vi "test - submodule case.vi"(8 "error in (no error)":errorcluster, 11 "TestCase in":refnum<class "csm-ini-variable-addon.lvclass">) -> (0 "error out":errorcluster, 3 "TestCase out":refnum<class "csm-ini-variable-addon.lvclass">)   [LabVIEW 2017, in "csm-ini-variable-addon.lvclass"]
uses:
  csm-ini-variable-addon.lvclass
  2c933430-14a5-474e-a898-733b1e5a1a8b.vi
  2c933430-14a5-474e-a898-733b1e5a1a8b.vi/99de0c97-112a-4c86-9094-c187659127e1.vi
  <userlib>/_NEVSTOP/Communicable State Machine(CSM)/Utility/Build Error Cluster.vi
  <vilib>/Utility/Data Type/Get Type Information.vi
  <userlib>/_NEVSTOP/Communicable State Machine(CSM)/addons/API-String-Arugments-Support/_Support/Data To SingleElementsArray_csm.vi
  <userlib>/_NEVSTOP/Communicable State Machine(CSM)/addons/API-String-Arugments-Support/_Support/Data To API String Arguments.vi
  INI-Static-Variable-Support/_Support/Parse Used Session and Name.vi
  INI-Static-Variable-Support/_Support/INI-FGV(lvlibp).vi
  INI-Static-Variable-Support/_Support/Populate String with INI Variable.vi
  <userlib>/_NEVSTOP/Communicable State Machine(CSM)/addons/API-String-Arugments-Support/_Support/Convert API String Arguments to Data(variant).vi
  <userlib>/_NEVSTOP/Communicable State Machine(CSM)/addons/API-String-Arugments-Support/_Support/SingleElementsArray To Data_csm.vi
  <vilib>/addons/_JKI Toolkits/VI Tester/TestCase.llb/TestCase.lvclass
  INI-Static-Variable-Support/INI-Static-Variable-Support.lvlib
  <userlib>/_NEVSTOP/Communicable State Machine(CSM)/addons/API-String-Arugments-Support/API String Arguments Support.lvlib
  C:/Program Files (x86)/National Instruments/LabVIEW 2017/vi.lib/addons/_JKI Toolkits/VI Tester/TestCase.llb/TestCase.lvclass
panel:
  out "String out":string
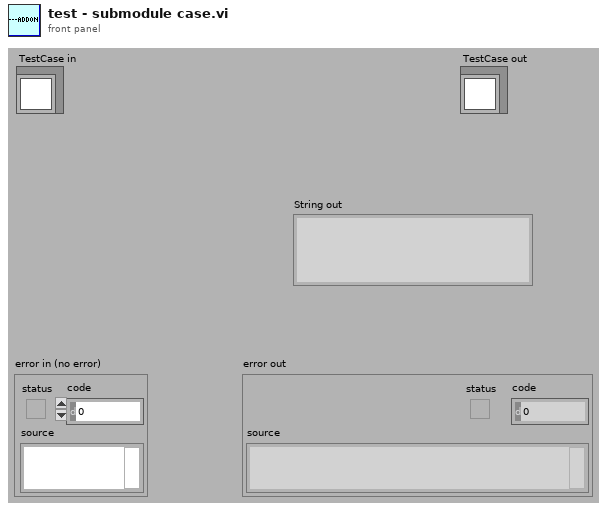
[diagram p1: front panel]
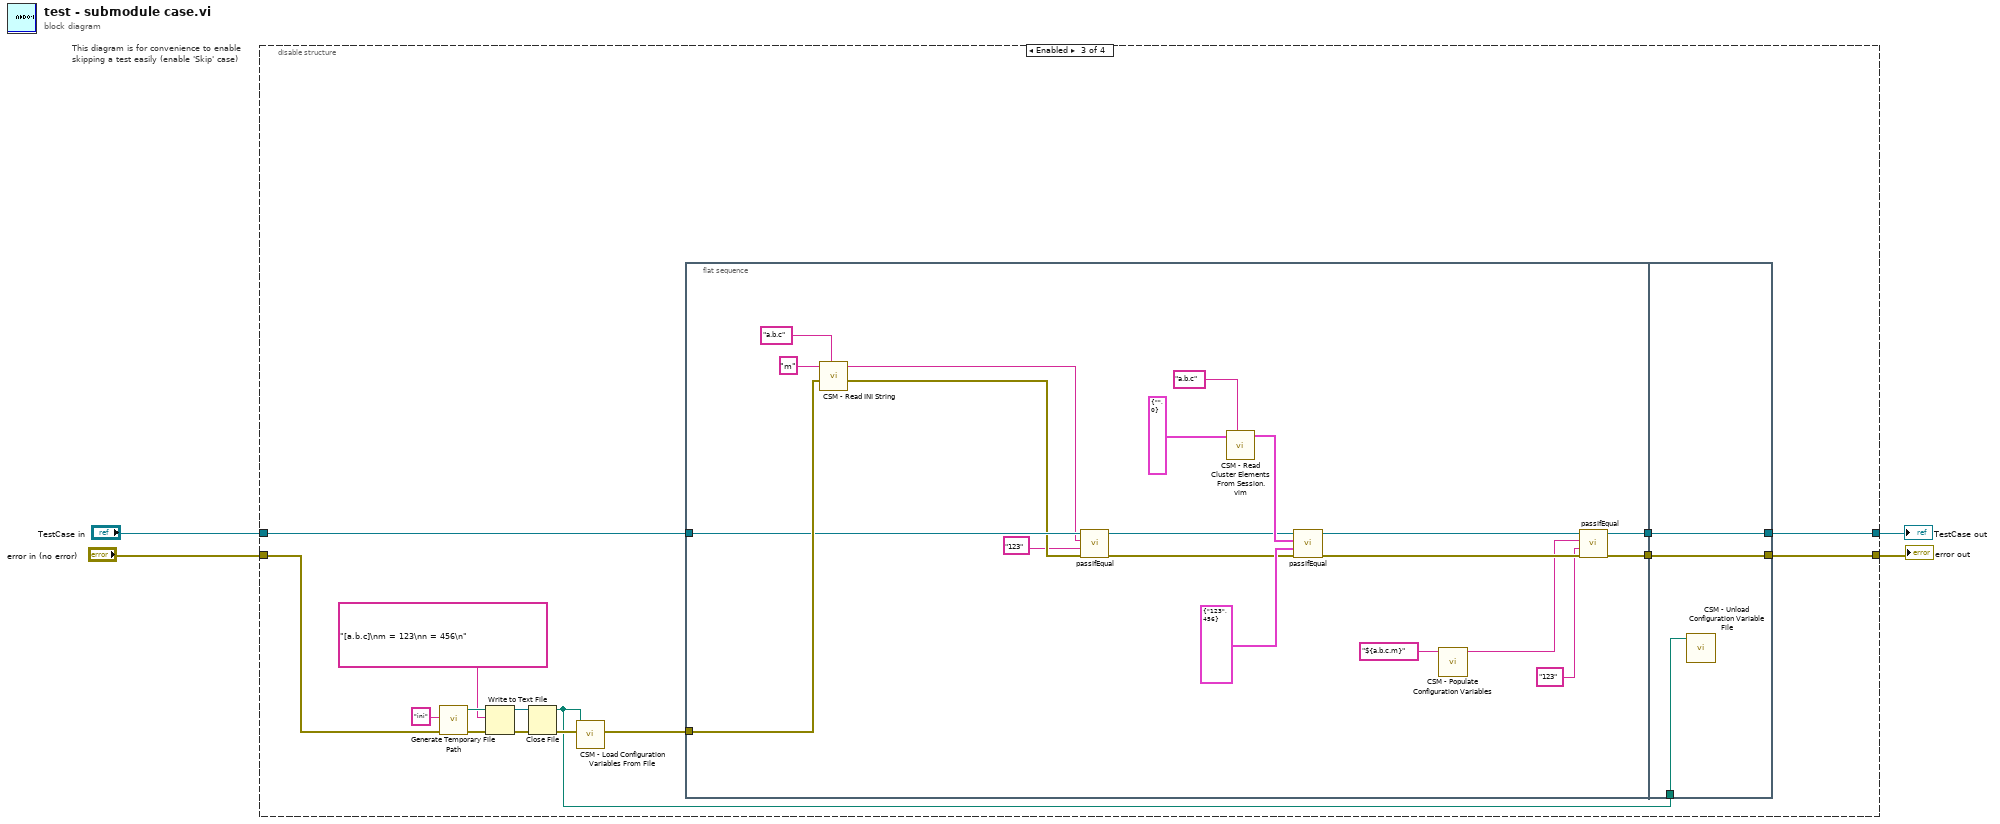
[diagram p0: block diagram]
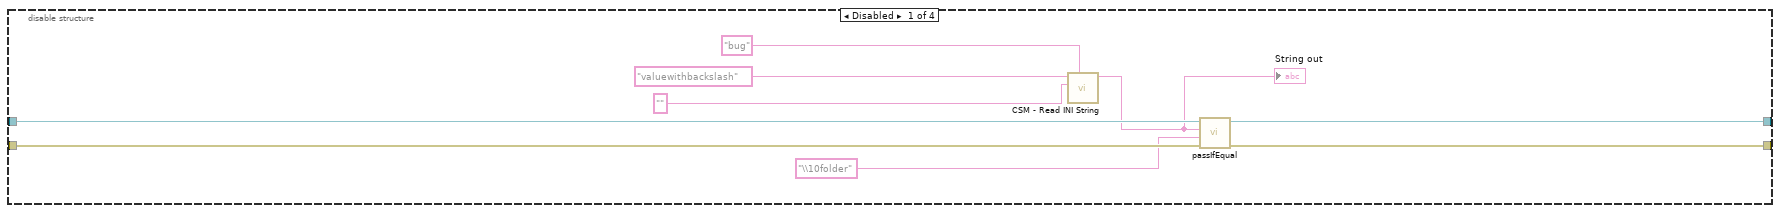
[diagram p2: hidden frame]
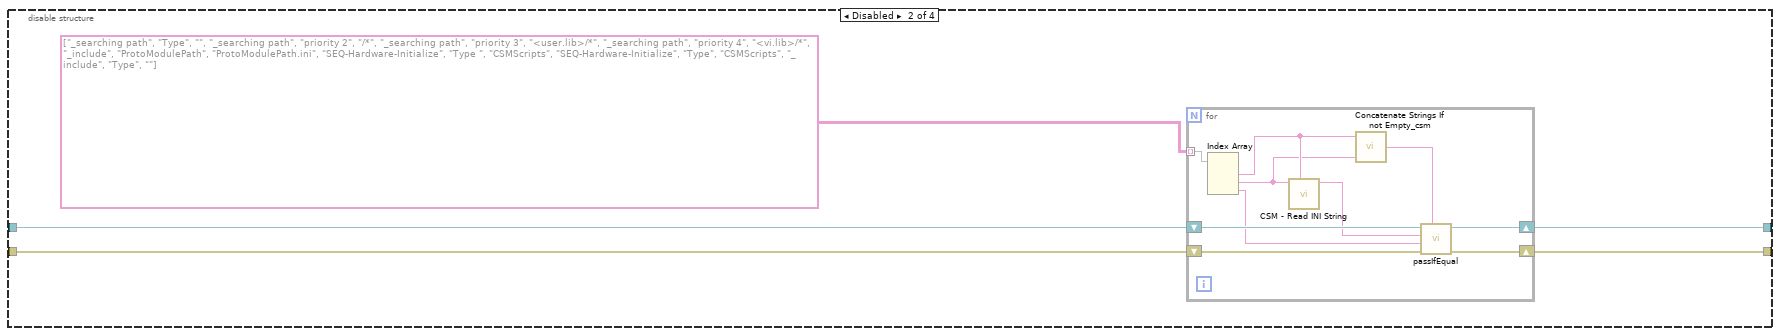
[diagram p3: hidden frame]
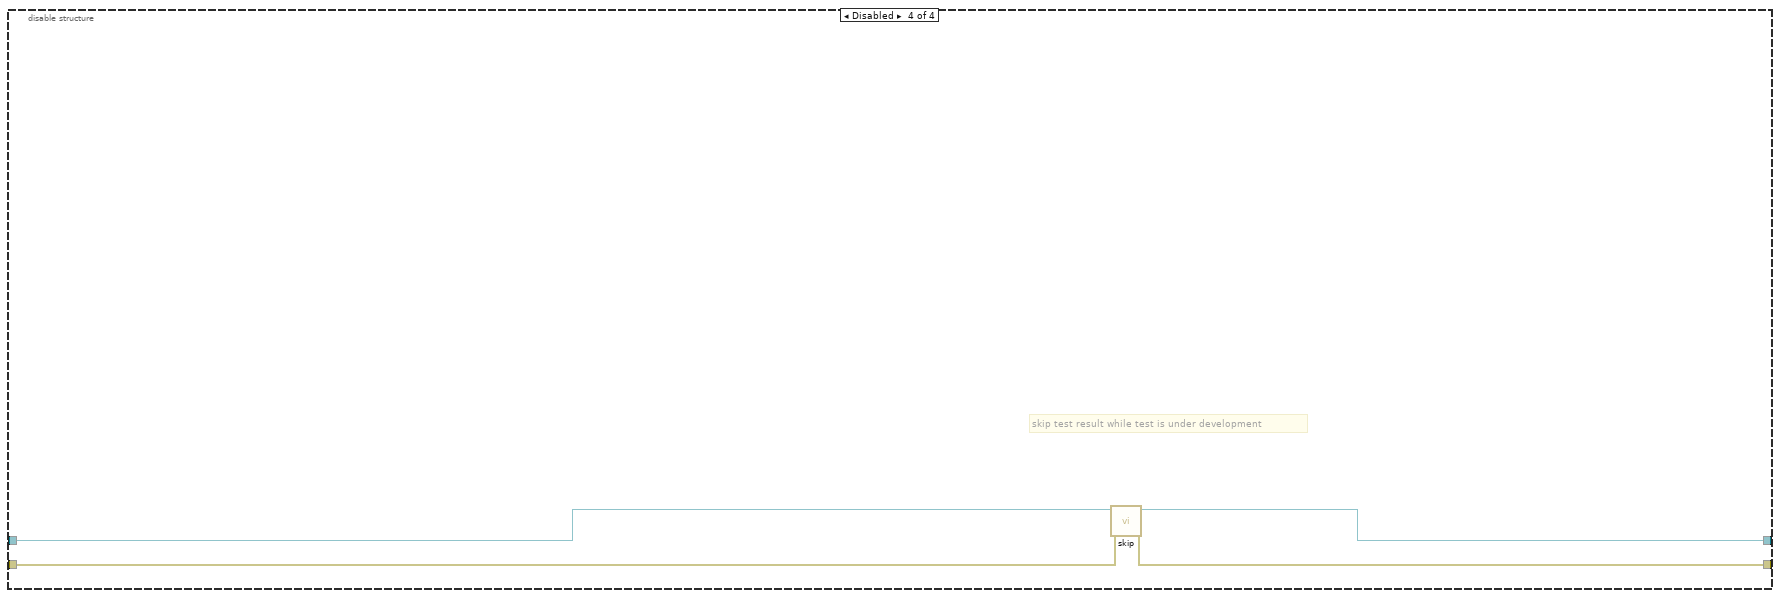
[diagram p4: hidden frame]
diagram:
  n1 = disable-structure "This diagram is for convenience to enable skipping a test easily (enable 'Skip' case)" shown="Enabled" {
    disable-tunnel: "TestCase in" -> [w10 w15 w34 w70]
    disable-tunnel: [w13 w18 w33 w68] -> w1
    disable-tunnel: [w12 w17 w32 w69] -> w3
    disable-tunnel: "error in (no error)" -> [w11 w16 w36 w67]
    frame Disabled {
      n2 = call "CSM - Read INI String.vi"("Section Name(\"\" as Default)"="bug" ("Section Name(\"\" as Default)"), ">> Default Value >>"="" ("String in"), "String in"="valuewithbackslash") -> ("String out"=w6:string)  [unwired: 4 in, 2 out]
      "String out" <- w6
      n3 = call-dynamic "passIfEqual.vi"("error in (no error)"=w11, "y"="\\10folder" ("String in"), "x"=w6, "TestCase in"=w10) -> ("error out"=w12:errorcluster, "TestCase out"=w13:refnum<class "csm-ini-variable-addon.lvclass">)  [unwired: 6 in]
    }
    frame Disabled {
      n4 = for {
        shift-right: [w27] -> w17
        shift-left: w16 -> [w26]
        shift-right: [w28] -> w18
        shift-left: w15 -> [w25]
        tunnel: string[][] [["_searching path", "Type", ""], ["_searching path", "priority 2", "/*"], ["_searching path", "priority 3", "<user.lib>/*"], ["_searching path", "priority 4", "<vi.lib>/*"], ["_include", "ProtoModulePath", "ProtoModulePath.ini"], ["SEQ-Hardware-Initialize", "Type ", "CSMScripts"], ["SEQ-Hardware-Initialize", "Type", "CSMScripts"], ["_include", "Type", ""]] -> [w23] mode=indexing
        n5 = Index Array(array=w23) -> (element #1=w20:string, element #2=w19:string, element #3=w22:string)  [unwired: 3 in]
        n6 = call "CSM - Read INI String.vi"("Section Name(\"\" as Default)"=w20, "String in"=w19) -> ("String out"=w24:string)  [unwired: 5 in, 2 out]
        n7 = call <userlib>:"Concatenate Strings If not Empty_csm.vi"("String"=w19, "prefix"=w20) -> ("result"=w21:string)  [unwired: 3 in]
        n8 = call-dynamic "passIfEqual.vi"("custom report message (\"\")"=w21, "error in (no error)"=w26, "y"=w22, "x"=w24, "TestCase in"=w25) -> ("error out"=w27:errorcluster, "TestCase out"=w28:refnum<class "csm-ini-variable-addon.lvclass">)  [unwired: 5 in]
      }
    }
    frame Enabled {
      n9 = call <vilib>:"Generate Temporary File Path.vi"("error in (no error)"=w36, "Temporary File Extension (tmp)"="ini") -> ("error out"=w43:errorcluster, "Unique Temporary File Path"=w40:path)  [unwired: 8 in]
      n10 = Write to Text File(file (use dialog)=w40, text="[a.b.c]\nm = 123\nn = 456\n", error in=w43) -> (refnum out=w39:refnum<file>, error out=w41:errorcluster)  [unwired: 1 in, 1 out]
      n11 = Close File(refnum=w39, error in=w41) -> (path=w29:path, error out=w38:errorcluster)
      n12 = call "CSM - Load Configuration Variables From File.vi"("error in (no error)"=w38, "Path"=w29) -> ("error out"=w35:errorcluster)  [unwired: 7 in]
      n13 = flat-sequence {
        tunnel: w35 -> [w63]
        tunnel: w34 -> [w62]
        tunnel: [w48] -> w31
        tunnel: [w47] -> w30
        tunnel: [w65] -> w32
        tunnel: [w66] -> w33
        tunnel: w31 -> [w66]
        tunnel: w30 -> [w65]
        tunnel: w29 -> [w64]
        frame #0 {
          n14 = call "CSM - Read INI String.vi"("Section Name(\"\" as Default)"="a.b.c" ("Section Name(\"\" as Default)"), "error in (no error)"=w63, "String in"="m") -> ("error out"=w61:errorcluster, "String out"=w58:string)  [unwired: 4 in, 1 out]
          n15 = call-dynamic "passIfEqual.vi"("error in (no error)"=w61, "y"="123" ("String in"), "x"=w58, "TestCase in"=w62) -> ("error out"=w50:errorcluster, "TestCase out"=w53:refnum<class "csm-ini-variable-addon.lvclass">)  [unwired: 6 in]
          n16 = call "CSM - Read Cluster Elements From Session.vim"("Section Name(\"\" as Default)"="a.b.c" ("Section Name(\"\" as Default)"), "Cluster"=cluster{"m":string, "n":i32} {"m"="", "n"=0}) -> ("Cluster out"=w54:cluster{"m":string, "n":i32})  [unwired: 6 in, 1 out]
          n17 = call-dynamic "passIfEqual.vi"("error in (no error)"=w50, "y"=cluster{"m":string, "n":i32} {"m"="123", "n"=456}, "x"=w54, "TestCase in"=w53) -> ("error out"=w51:errorcluster, "TestCase out"=w49:refnum<class "csm-ini-variable-addon.lvclass">)  [unwired: 6 in]
          n18 = call "CSM - Populate Configuration Variables.vi"("String in"="${a.b.c.m}") -> ("String out"=w45:string)  [unwired: 7 in, 1 out]
          n19 = call-dynamic "passIfEqual.vi"("error in (no error)"=w51, "y"="123" ("String in"), "x"=w45, "TestCase in"=w49) -> ("error out"=w47:errorcluster, "TestCase out"=w48:refnum<class "csm-ini-variable-addon.lvclass">)  [unwired: 6 in]
        }
        frame #1 {
          n20 = call "CSM - Unload Configuration Variable File.vi"("Path"=w64) -> ()  [unwired: 8 in, 1 out]
        }
      }
    }
    frame Disabled {
      # "skip test result while test is under development"
      n21 = call <vilib>:"skip.vi"("error in (no error)"=w67, "TestCase in"=w70) -> ("error out"=w69:errorcluster, "TestCase out"=w68:refnum<class "csm-ini-variable-addon.lvclass">)  [unwired: 8 in]
    }
  }
  "error out" <- w3
  "TestCase out" <- w1
